vi "BUILD_vipb path.vi"() -> (3 "appended path":path)   [LabVIEW 2013]
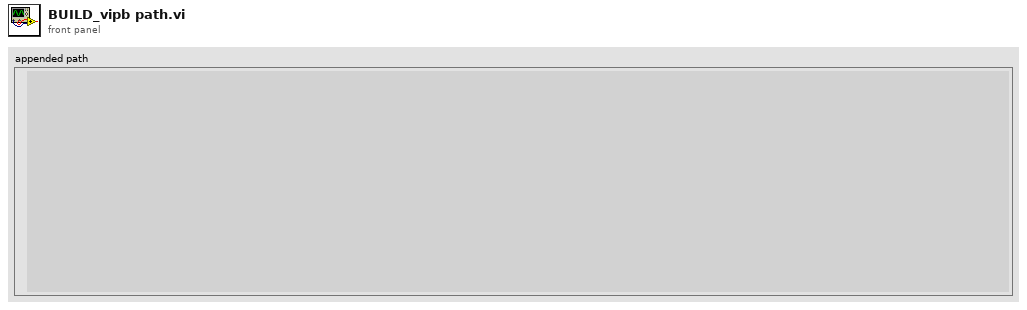
[diagram p1: front panel]
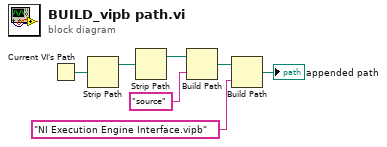
[diagram p0: block diagram]
diagram:
  n1 = Current VI's Path() -> (path=w1:path)
  n2 = Strip Path(path=w1) -> (stripped path=w2:path)  [unwired: 1 out]
  n3 = Strip Path(path=w2) -> (stripped path=w4:path)  [unwired: 1 out]
  n4 = Build Path(base path=w4, name or relative path="source") -> (appended path=w6:path)
  n5 = Build Path(base path=w6, name or relative path="NI Execution Engine Interface.vipb") -> (appended path=→"appended path":path)
